vi "Map Dilico Voltages.vi"(10 "#Cell Request":u8=10 max=96, 11 "CAN Frame Input":T1[](array[typedef]) {"payload" format="%x"; "timestamp" format="%<%.7X\n%x>T"; "type" items=["CAN Data"=0, "CAN Remote"=1, "CAN Bus Error"=2, "CAN 2.0 Data"=8, "CAN FD Data"=16, "CAN FD+BRS Data"=24, "J1939 Data"=192, "Delay"=224, "Log Trigger"=225, "Start Trigger"=226]; "identifier" format="%x"}) -> (3 "Dilico Values":map{string, dbl}(c390))   [LabVIEW 2025, in "phlair-busch-can-bus.lvlib"]
uses:
  phlair-busch-can-bus.lvlib
  <vilib>/xnet/xnet.llb/XNET Frame CAN.ctl
  <vilib>/xnet/xnet.llb/XNET Frame Type CAN.ctl
panel:
  out "CVM":cluster{i32[], dbl[unit][]}
  out "Sum Cells":dbl[unit] format="%#_6p"
  out "Frames received":i32
  out "Cell[i] mV":dbl[unit][](array[numeric])
  out "Cell Index":u8[](array[numeric])
  out "Index UV/OV":u8[](array[numeric]) format="%.0x"
  out "UV/OV raw data":u8[](array[numeric]) format="%.0x"
  # "Input"
  # "Inner"
  # "Output"
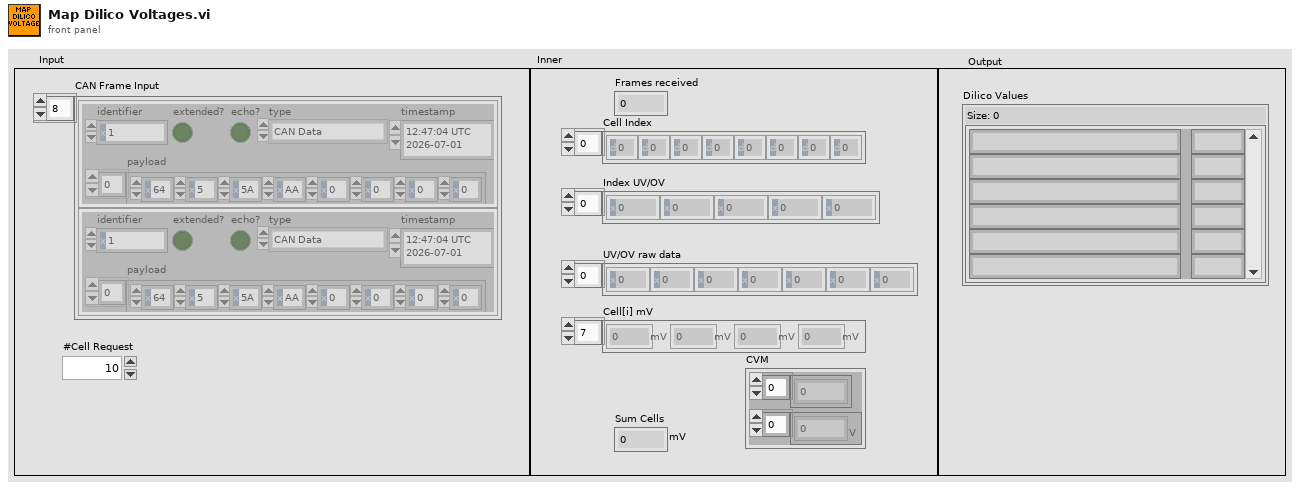
[diagram p1: front panel]
types:
  T1 = typedef "XNET Frame CAN.ctl" = cluster{"timestamp":timestamp, "payload":u8[], "identifier":u32, "type":T2, "extended?":bool, "echo?":bool}
  T2 = typedef "XNET Frame Type CAN.ctl" = u8
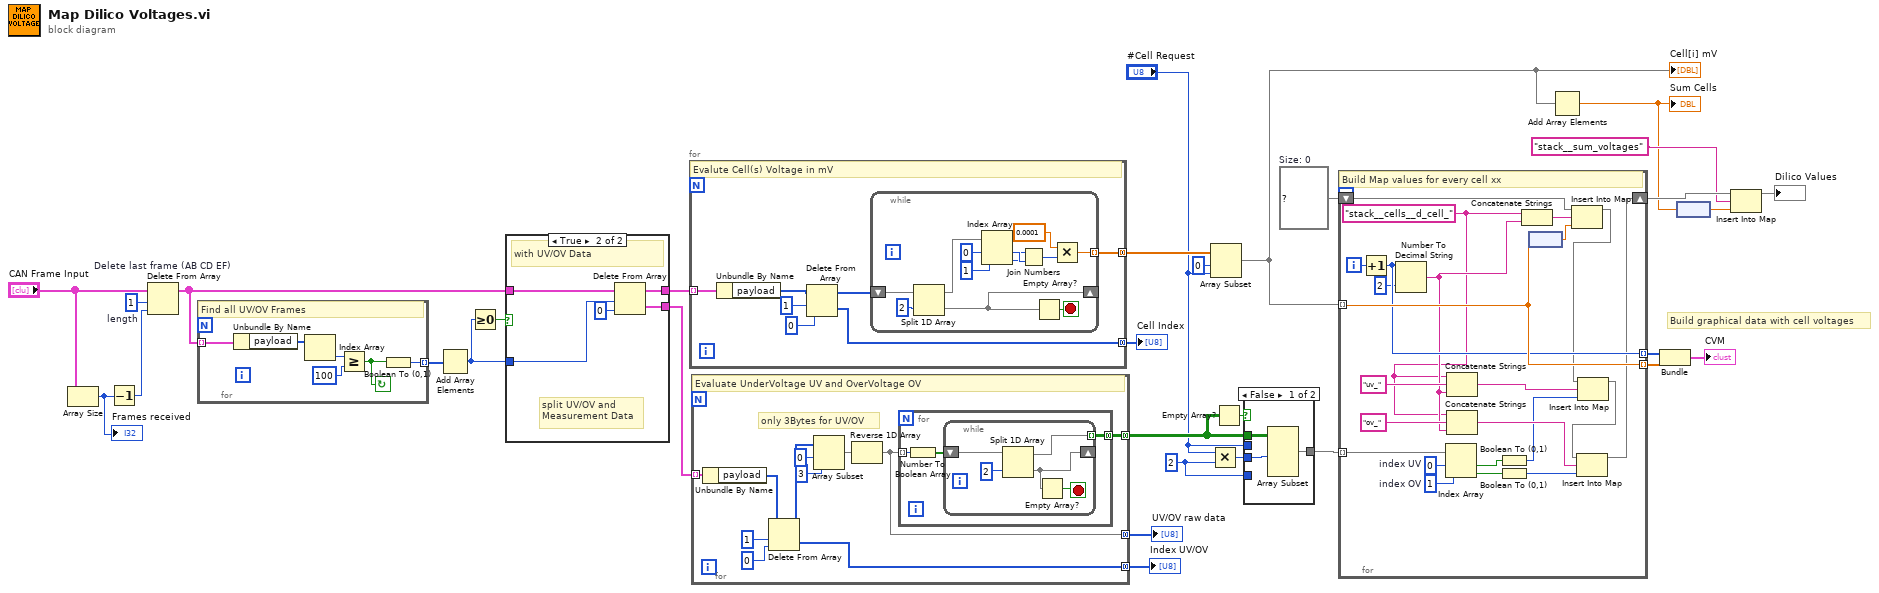
[diagram p0: block diagram]
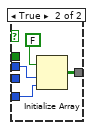
[diagram p2: hidden frame]
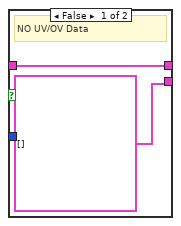
[diagram p3: hidden frame]
diagram:
  w17 = map{string, dbl} {}  # Size: 0
  w7 = u8 2 ("y")
  w25 = 1  # length
  # "Build graphical data with cell voltages"
  n1 = Array Size(array="CAN Frame Input") -> (size(s)=w26:i32)
  "Frames received" <- w26
  n2 = Decrement(x=w26) -> (x-1=w24:i32)
  n3 = Delete From Array "Delete last frame (AB CD EF)"(array="CAN Frame Input", length=w25, index=w24) -> (array with subset deleted=w3:T1[])  [unwired: 1 out]
  n4 = for {
    tunnel: w3 -> [w37] mode=indexing
    tunnel: [w32] -> w4 mode=indexing
    stop <- w33 continue-if-true
    # "Find all UV/OV Frames"
    n5 = Unbundle By Name(w37) -> ("payload"=w36:u8[])
    n6 = Index Array(array=w36) -> (element=w35:u8)  [unwired: 1 in]
    n7 = Greater Or Equal?(x=w35, y=u8 100) -> (x >= y?=w33:bool)
    n8 = Boolean To (0,1)(Boolean=w33) -> (0, 1=w32:i16)
  }
  n9 = Add Array Elements(numeric array=w4) -> (sum=w1:i16)
  n10 = Greater Or Equal To 0?(x=w1) -> (x >= 0?=w2:bool)
  n11 = case shown="True" w2 {
    tunnel: [T1[] [] ("CAN Frame Input") w44] -> w31
    tunnel: [w39 w42] -> w28
    tunnel: w3 -> [w39 w41]
    tunnel: w1 -> [_ w40]
    frame False {
      # "NO UV/OV Data"
    }
    frame True {
      # "split UV/OV and\nMeasurement Data"
      # "with UV/OV Data"
      n12 = Delete From Array(array=w41, length=w40, index=0) -> (deleted portion=w44:T1[], array with subset deleted=w42:T1[])
    }
  }
  n13 = for {
    tunnel: w28 -> [w51] mode=indexing
    tunnel: [w47] -> w27 mode=concatenating
    tunnel: [w45] -> w21 mode=concatenating
    # "Evalute Cell(s) Voltage in mV"
    n14 = Unbundle By Name(w51) -> ("payload"=w48:u8[])
    n15 = Delete From Array(array=w48, length=1, index=0) -> (deleted portion=w47:u8[], array with subset deleted=w46:u8[])
    n16 = while {
      shift-right: [w60] -> _
      shift-left: w46 -> [w63]
      tunnel: [w52] -> w45 mode=indexing
      stop <- w62 stop-if-true
      n17 = Split 1D Array(array=w63, index=2) -> (first subarray=w57:u8[], second subarray=w60:u8[])
      n18 = Index Array(array=w57, index #1=0 ("index"), index #2=1 ("index")) -> (element #1=w56:u8, element #2=w55:u8)
      n19 = Join Numbers(hi=w55, lo=w56) -> ((hi.lo)=w53:u16)
      n20 = Empty Array?(array=w60) -> (empty?=w62:bool)
      n21 = Multiply(x=dbl[unit] 0.0001, y=w53) -> (x*y=w52:dbl[unit])
    }
  }
  "Cell Index" <- w27
  n22 = for {
    tunnel: w31 -> [w74] mode=indexing
    tunnel: [w71] -> w29 mode=concatenating
    tunnel: [w72] -> w30 mode=concatenating
    tunnel: [w70] -> w9 mode=concatenating
    # "only 3Bytes for UV/OV"
    # "Evaluate UnderVoltage UV and OverVoltage OV"
    n23 = Unbundle By Name(w74) -> ("payload"=w68:u8[])
    n24 = Delete From Array(array=w68, length=1, index=0) -> (deleted portion=w72:u8[], array with subset deleted=w66:u8[])
    n25 = Array Subset(array=w66, index=0, length=3) -> (w67:u8[])
    n26 = Reverse 1D Array(array=w67) -> (reversed array=w71:u8[])
    n27 = for {
      tunnel: w71 -> [w77] mode=indexing
      tunnel: [w76] -> w70 mode=concatenating
      n28 = Number To Boolean Array(number=w77) -> (Boolean array=w75:bool[])
      n29 = while {
        shift-right: [w80] -> _
        shift-left: w75 -> [w82]
        tunnel: [w78] -> w76 mode=indexing
        stop <- w81 stop-if-true
        n30 = Split 1D Array(array=w82, index=2) -> (first subarray=w78:bool[], second subarray=w80:bool[])
        n31 = Empty Array?(array=w80) -> (empty?=w81:bool)
      }
    }
  }
  "UV/OV raw data" <- w29
  "Index UV/OV" <- w30
  n32 = Multiply(x="#Cell Request", y=w7) -> (x*y=w19:u8)
  n33 = Array Subset(array=w21, index=0, length="#Cell Request") -> (w18:dbl[unit][])
  "Cell[i] mV" <- w18
  n34 = Empty Array?(array=w9) -> (empty?=w8:bool)
  n35 = case shown="False" w8 {
    tunnel: [w85 w89] -> w20
    tunnel: w19 -> [w84 _]
    tunnel: w9 -> [w83 _]
    tunnel: w7 -> [_ w86]
    tunnel: "#Cell Request" -> [_ w87]
    frame False {
      n36 = Array Subset(array=w83, length (row)=w84) -> (w85:bool[][])  [unwired: 3 in]
    }
    frame True {
      n37 = Initialize Array(FALSE, w87, w86) -> (w89:bool[][])
    }
  }
  n38 = for {
    tunnel: w18 -> [w109] mode=indexing
    tunnel: w20 -> [w107] mode=indexing
    shift-right: [w96] -> w16
    shift-left: w17 -> [w111]
    tunnel: [w109] -> w11 mode=indexing
    tunnel: [w108] -> w12 mode=indexing
    i -> [w112]
    w105 = 1  # index OV
    w106 = 0  # index UV
    w93 = "stack__cells__d_cell_"
    # "Build Map values for every cell xx"
    n39 = Increment(x=w112) -> (x+1=w108:i32)
    n40 = Number To Decimal String(number=w108, width (-)=i16 2) -> (decimal integer string=w94:string)
    n41 = Index Array(array=w107, index #1=w106, index #2=w105) -> (element #1=w91:bool, element #2=w103:bool)
    n42 = Concatenate Strings(w93, "uv_" ("key"), w94) -> (w100:string)
    n43 = Concatenate Strings(w93, "ov_" ("key"), w94) -> (w99:string)
    n44 = Boolean To (0,1)(Boolean=w91) -> (0, 1=w95:i16)
    n45 = Boolean To (0,1)(Boolean=w103) -> (0, 1=w90:i16)
    n46 = Concatenate Strings(w93, w94) -> (w101:string)
    n47 = node(w109) -> (w110:dbl)
    n48 = Insert Into Map(map in=w111, key=w101, value=w110) -> (map out=w98:map{string, dbl})  [unwired: 2 out]
    n49 = Insert Into Map(map in=w98, key=w100, value=w95) -> (map out=w97:map{string, dbl})  [unwired: 2 out]
    n50 = Insert Into Map(map in=w97, key=w99, value=w90) -> (map out=w96:map{string, dbl})  [unwired: 2 out]
  }
  n51 = Add Array Elements(numeric array=w18) -> (sum=w14:dbl[unit])
  "Sum Cells" <- w14
  n52 = Bundle(w12, w11) -> (→"CVM":cluster{i32[], dbl[unit][]})  [unwired: 1 in]
  n53 = node(w14) -> (w13:dbl)
  n54 = Insert Into Map(map in=w16, key="stack__sum_voltages", value=w13) -> (map out=→"Dilico Values":map{string, dbl})  [unwired: 2 out]
